vi "InitializeInstrument.vi"(8 "error in (no error)":errorcluster, 11 "reference in":refnum<class "niMmWave_Reciever.lvclass">) -> (0 "error out":errorcluster, 3 "reference out":refnum<class "niMmWave_Reciever.lvclass">)   [LabVIEW 2019, in "niMmWave_Reciever.lvclass"]
doc: "Opens instrument session(s) and performs initial configuration for selected mode.\n\nInputs:\n<b>Initialization source</b> ini file and ini section to be read\n<b>Mode</b> specifies operation mode: BB/IF/RF"
uses:
  niMmWave_Reciever.lvclass
  C:/Barkhausen mmWave radar/Development/modules/mmw_instrument/src_LabVIEW/Host/SubVIs/mmWave instrument_class/mmWave instrument.lvclass
  Low-level/TypeDefs/Resources.ctl
  <vilib>/userdefined/High Color/nirio_resource_hc.ctl
  mmWave instrument_class/Instrument state.ctl
  Low-level/TypeDefs/Hardware Configuration.ctl
  Low-level/TypeDefs/Direction.ctl
  mmWave HW Control/mmWave HW Control.lvlib
  mmWave instrument_class/mmWave instrument.lvclass
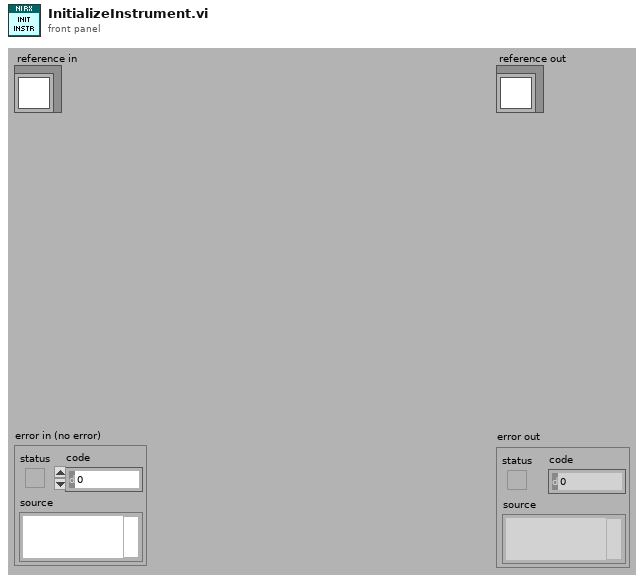
[diagram p1: front panel]
types:
  T1 = typedef "mmWave instrument.lvclass/Instrument state.ctl" = enum16{"Off", "Initialization", "Configuration", "Running", "Calibration"}
  T2 = typedef "Resources.ctl" = cluster{"7902R (Tx)":T3, "3610 (Tx)":refnum<visa-resource-name>, "3620 (IF)":T3, "3630 (RX)":refnum<visa-resource-name>, "7902R (Rx)":T3}
  T3 = typedef "nirio_resource_hc.ctl" = tag
  T4 = typedef "mmWave instrument.lvclass/ObjectAttributesRef.ctl" = refnum<data-value>
  T5 = typedef "niMmWave_Reciever.lvclass/ObjectAttributesRef.ctl" = refnum<data-value>
  T6 = typedef "niMmWave_Reciever.lvclass/ObjectAttributes.ctl" = cluster{"session":T7[], "HW.RX devices":T21, "RF config":T22, "RX trigger options":T23, "RX samples":i32, "RX Fs":dbl}
  T7 = typedef "Session.ctl" = cluster{"3620 session":refnum<queue>, "tx baseband session":T8, "rx baseband session":T16, "tx gain (dB)":dbl, "rx gain (dB)":dbl, "hardware configuration":T17, "gain ranging":T19[], "pxi trigger bus information":T20}
  T8 = typedef "Tx Baseband Session.ctl" = cluster{"3610 session":T9, "7902 reference":T15}
  T9 = typedef "ni3610_and_ni3630_Driver_Lib.lvlib/Main Settings.ctl" = cluster{"VISA resource name":refnum<visa-resource-name>, "Address Space":T10, "window_offset":u32, "register_addresses":T11, "required_MM_fpga_version":cluster{"signature":u32, "hardware":u32, "current revision":u32, "oldest revision":u32}, "CPLD Oldest Compat Version ":cluster{"hardware":u32, "CPLD firmware":u32}, "MM_FPGA_image_location":string, "is_init":bool, "card_type":T12, "DacLmkConfigFileName":string, "AdcLmkConfigFileName":string, "AdcConfigFileName":string, "DacConfigFileName_RevA":string, "DacConfigFileName_RevB":string, "Mulde hardware revision":u8, "bypass DAC PLL\n":bool, "IQ Card Revision":T13, "board capability":T14}
  T10 = typedef "VISA Register Access Address Space.ctl" = u16
  T11 = typedef "ni3610_and_ni3630_Driver_Lib.lvlib/Register Adresses.ctl" = cluster{"MM based Registers":cluster{"Revision":u32, "OldestCompatRev":u32, "signature":u32, "scratch":u32, "LedControl":u32, "BoardHwRev":u32, "BoardControl":u32, "ThermalStatus":u32, "BasebandStatus":u32, "BasebandControl":u32, "BasebandAuxSetup":u32, "BasebandAuxStatus":u32, "LmkSyncOutSetup":u32, " AdcSyncOutSetup":u32, " InjSyncOutSetup":u32, " PxiTrig0OutSetup":u32, " PxiTrig1OutSetup":u32, " PxiTrig2OutSetup":u32, " PxiTrig3OutSetup":u32, " PxiTrig4OutSetup":u32, " PxiTrig5OutSetup":u32, " PxiTrig6OutSetup":u32, " PxiTrig7OutSetup":u32}, "CPLD based Registers":cluster{"SlaveSignature":u32, "SlaveRevision":u32, "SlaveOldestCompatRev":u32, "SlaveScratch":u32, "SlaveSetup":u32, "SlaveStatus":u32, "IDacReg_offset":u32, "LMKRegGrp0_offset":u32, "QDacReg_offset":u32, "BrdTempSensorVal":u32, "TempSensorPowerDown":u32, "GPIOReg_offset":u32, "IAdcReg_offset":u32, "QAdcReg_offset":u32, "LMKRegGrp1_offset":u32, "QadcTempSensorVal":u32, "IadcTempSensorVal":u32, "RevisionReg":u32, "VcxoReg":u32, "CpldStatusReg":u32, "PowerReg":u32, "VBiasEnReg":u32, "ExtRefOeReg":u32, "QdacCtrlReg":u32, "QdacStatusReg":u32, "IdacCtrlReg":u32, "IdacStatusReg":u32, "QdacJtagIn":u32, "QdacJtagOut":u32, "IdacJtagIn":u32, "IdacJtagOut":u32, "IqDcSetupReg":u32, "QadcStatusReg":u32, "IadcStatusReg":u32, "BrdSetupReg":u32, "IqDcRevisionReg":u32, "PllStatusReg":u32, "EndpointScratchReg":u32, "AdcSyncCfgReg":u32, "IqCardOpampReg":u32}, "CPLD Register Offset":u32, "MM  Register Offset":u32, " PxiTrig0OutSetup":u32}
  T12 = typedef "ni3610_and_ni3630_Driver_Lib.lvlib/Base Card Type.ctl" = enum16{"unspecified", "ADC", "DAC"}
  T13 = typedef "ni3610_and_ni3630_Driver_Lib.lvlib/IQ Card Revision.ctl" = enum16{"RevA", "RevB", "RevC", "RevD"}
  T14 = typedef "ni3610_and_ni3630_Driver_Lib.lvlib/Board Capability.ctl" = cluster{"baseband sync":enum16{"no baseband sync", "baseband sync"}}
  T15 = typedef "Blank FPGA Reference.ctl" = refnum<k20>
  T16 = typedef "Rx Baseband Session.ctl" = cluster{"3630 session":T9, "7902 reference":T15}
  T17 = typedef "Hardware Configuration.ctl" = cluster{"direction":T18, "baseband only":bool}
  T18 = typedef "Direction.ctl" = enum16{"Transceiver", "Receiver", "Transmitter"}
  T19 = typedef "Gain Ranging.ctl" = cluster{"gain ranging active scope":string, "gain ranging stream session":refnum<k20>}
  T20 = typedef "PXI Trigger Bus Info.ctl" = cluster{"chassis resource name":refnum<visa-resource-name>, "7902R (TX)":i16, "3610 (TX)":i16, "3620 (IF)":i16, "3630 (RX)":i16, "7902R (RX)":i16}
  T21 = typedef "mmWave HW Control.lvlib/HW RX resources cluster.ctl" = cluster{"HW.IF":tag, "HW.ADC":refnum<visa-resource-name>, "HW.RX FPGA":tag}
  T22 = typedef "mmWave HW Control.lvlib/HW RX RF config cluster.ctl" = cluster{"Gain":dbl, "Frequency":dbl, "mmWave adapter":string}
  T23 = typedef "TX trigger config.ctl" = cluster{"delay":dbl, "trig source":T24, "PXI src":i32, "export":T25, "PXI dest":i32}
  T24 = typedef "FPGA Utility.lvlib/FPGA driver trigger source.ctl" = enum16{"Use Tclk", "PXI_Trig", "Aurora RX trig"}
  T25 = typedef "FPGA Utility.lvlib/FPGA driver trigger destination.ctl" = enum16{"None", "Source trig", "Synced trig", "Delayed sync"}
  T26 = typedef "mmWave instrument.lvclass/ObjectAttributes.ctl" = cluster{"mode":T27, "instr state":T1, "Max Fs":dbl, "Equalization coeff":cdb[], "LO sync en":bool, "Trig sync en":bool, "LO sources":T28, "LO Export":T29, "Fc.range":cluster{"min":dbl, "max":dbl}, "Sync mode":T30, "equalization en":bool, "sequence":string[]}
  T27 = typedef "mmWave instrument.lvclass/Instrument mode.ctl" = enum16{"RF", "IF", "BB"}
  T28 = typedef "mmWave HW Control.lvlib/LO sources.ctl" = cluster{"RX/LO1 src":string, "TX/LO1 src":string, "LO2 src":string}
  T29 = typedef "mmWave HW Control.lvlib/LO export.ctl" = cluster{"TX LO1 export":bool, "TX LO1 export level":dbl, "RX LO1 export":bool, "RX LO1 export level":dbl, "LO2 export":bool, "LO2 export level":dbl}
  T30 = typedef "mmWave instrument.lvclass/Sync mode.ctl" = enum16{"Slave", "Master"}
  T31 = typedef "Detected mmWave Adapters.ctl" = cluster{"3620 resource name":T3, "detected mmWave adapters":T32[]}
  T32 = typedef "mmWave Adapter Information.ctl" = cluster{"scope":string, "mmWave adapter type":string, "serial number":u64}
  T33 = typedef "Constants.ctl" = cluster{"data clock rate (Hz)":dbl, "sample rate (Hz)":dbl, "sample rate selector string":string, "default tx bitfile path":path, "default rx bitfile path":path, "default proc bitfile path":path}
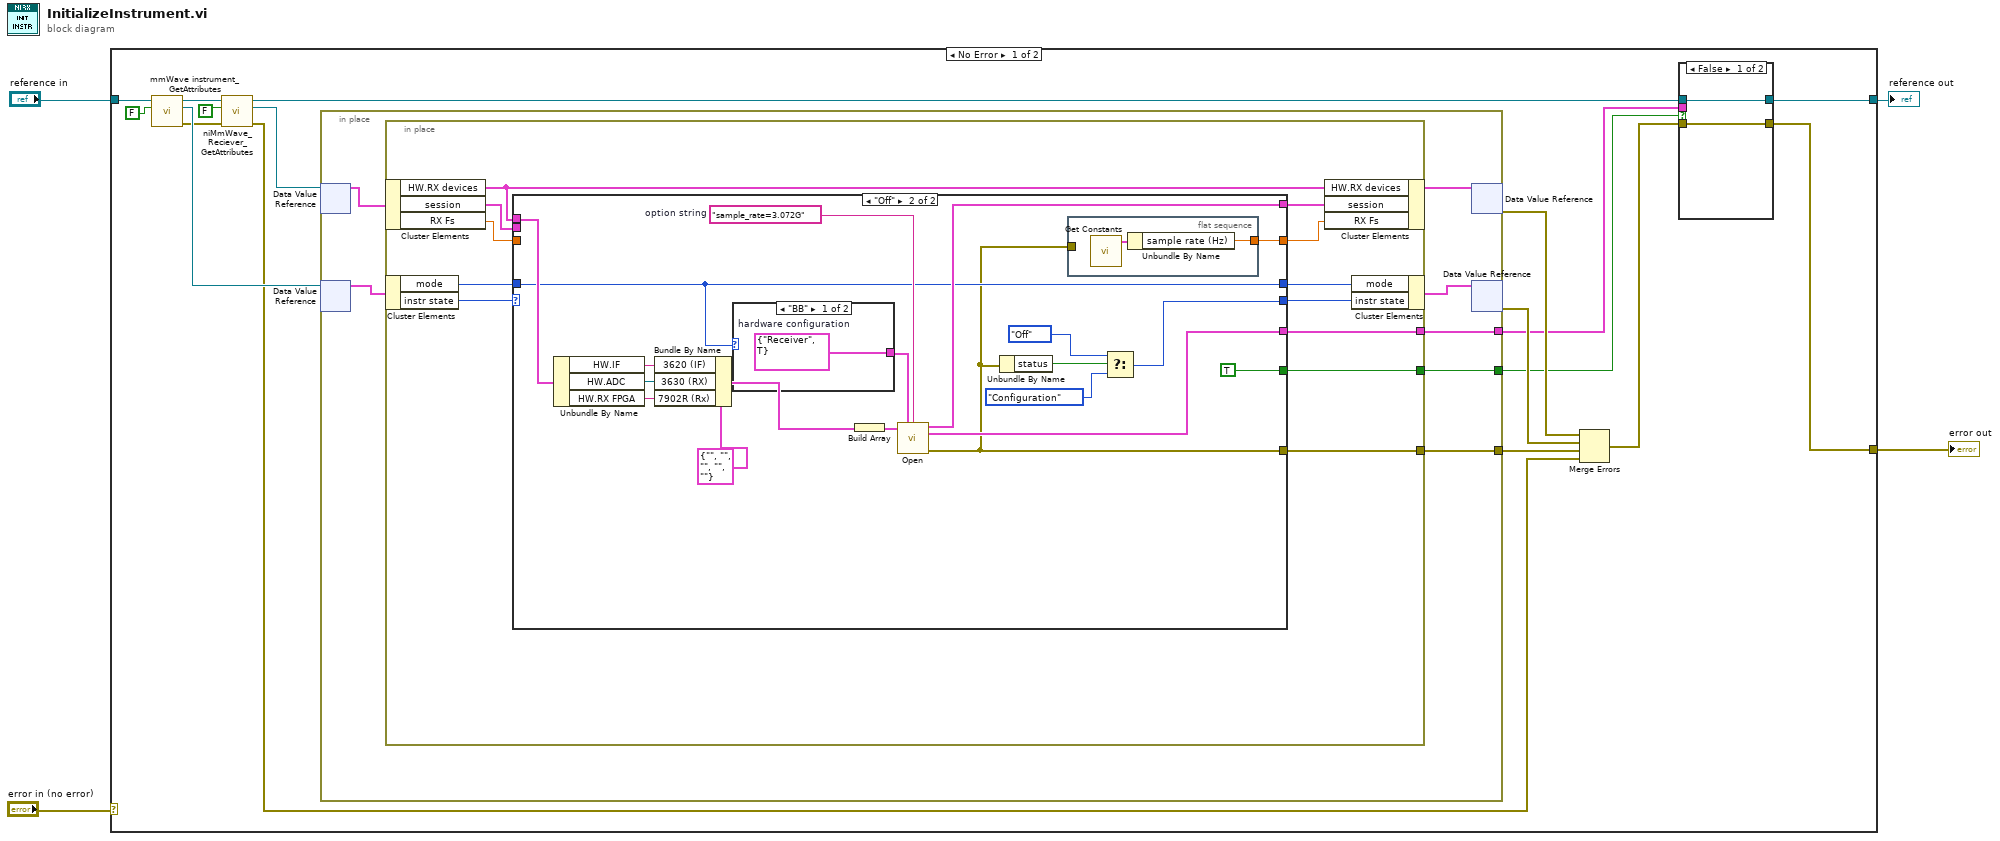
[diagram p0: block diagram]
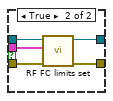
[diagram p2: hidden frame]
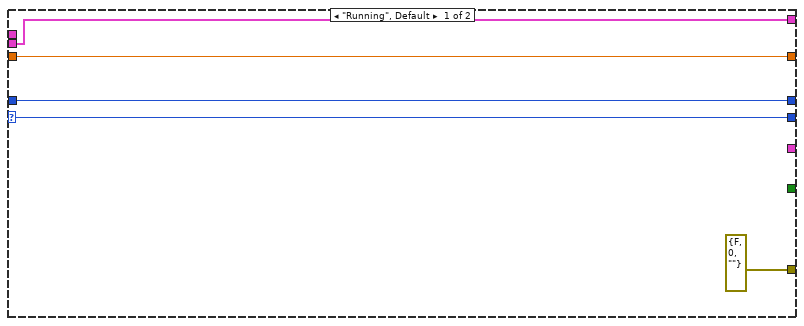
[diagram p3: hidden frame]
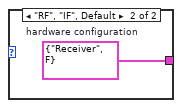
[diagram p4: hidden frame]
diagram:
  n1 = case shown="No Error" "error in (no error)" {
    selector: "error in (no error)" -> [_ w77]
    tunnel: [w6 w77] -> w3
    tunnel: [w9 w76] -> w1
    tunnel: "reference in" -> [w20 w76]
    frame No Error {
      n2 = call "mmWave instrument_GetAttributes.vi"("return data? (T)"=FALSE, "reference in"=w20) -> ("error out"=w13:errorcluster, "attributes ref"=w15:T4, "reference out"=w19:refnum<class "niMmWave_Reciever.lvclass">)  [unwired: 6 in, 1 out]
      n3 = call "niMmWave_Reciever_GetAttributes.vi"("error in (no error)"=w13, "return data? (T)"=FALSE, "reference in"=w19) -> ("error out"=w10:errorcluster, "attributes ref"=w16:T5, "reference out"=w21:refnum<class "niMmWave_Reciever.lvclass">)  [unwired: 5 in, 1 out]
      n4 = in-place {
        in-place-border: [w31] -> w14
        in-place-border: [w30] -> w8
        in-place-border: [w29] -> w5
        n5 = in-place-dvr #1(w16) -> (w35:T6)  [unwired: 1 out]
        n6 = in-place-dvr #2(w15) -> (w33:T26)  [unwired: 1 out]
        n7 = in-place {
          in-place-border: [w44] -> w31
          in-place-border: [w38] -> w30
          in-place-border: [w37] -> w29
          n8 = in-place-cluster #3(w35) -> ("HW.RX devices"=w47:T21, "session"=w36:T7[], "RX Fs"=w39:dbl)
          n9 = in-place-cluster #4(w33) -> ("mode"=w45:T27, "instr state"=w42:T1)
          n10 = case shown="\"Off\"" w42 {
            selector: w42 -> [w48 _]
            tunnel: w47 -> [_ w64]
            tunnel: [w49 w63] -> w46
            tunnel: w45 -> [w52 w57]
            tunnel: [errorcluster {"status"=FALSE, "code"=0, "source"=""} ("error out") w53] -> w44
            tunnel: [w48 w58] -> w43
            tunnel: [w52 w57] -> w41
            tunnel: [w50 w56] -> w40
            tunnel: w39 -> [w50 _]
            tunnel: [_ w55] -> w38
            tunnel: [_ TRUE] -> w37
            tunnel: w36 -> [w49 _]
            frame "Running", Default {
            }
            frame "Off" {
              w65 = "sample_rate=3.072G"  # option string
              n11 = Unbundle By Name(w64) -> ("HW.IF"=w69:tag, "HW.ADC"=w68:refnum<visa-resource-name>, "HW.RX FPGA"=w67:tag)
              n12 = Bundle By Name(cluster=T2 {"7902R (Tx)"="", "3610 (Tx)"="", "3620 (IF)"="", "3630 (RX)"="", "7902R (Rx)"=""} ("resources"), "3620 (IF)"=w69, "3630 (RX)"=w68, "7902R (Rx)"=w67) -> (w71:T2)
              n13 = case shown="\"BB\"" w57 {
                tunnel: [w74 w75] -> w62
                frame "BB" {
                  w74 = T17 {"direction"=enum."Receiver", "baseband only"=TRUE}  # hardware configuration
                }
                frame "RF", "IF", Default {
                  w75 = T17 {"direction"=enum."Receiver", "baseband only"=FALSE}  # hardware configuration
                }
              }
              n14 = Build Array(w71) -> (w70:T2[])
              n15 = call "Open.vi"("resources"=w70, "hardware configuration"=w62, "option string"=w65) -> ("session out"=w63:T7[], "detected mmWave adapters"=w55:T31[], "error out"=w53:errorcluster)  [unwired: 10 in]
              n16 = Unbundle By Name(w53) -> ("status"=w61:bool)
              n17 = flat-sequence {
                tunnel: [w73] -> w56
                tunnel: w53 -> [_]
                frame #0 {
                  n18 = call "Get Constants.vi"() -> ("constants"=w72:T33)  [unwired: 15 in]
                  n19 = Unbundle By Name(w72) -> ("sample rate (Hz)"=w73:dbl)
                }
              }
              n20 = Select(t=Instrument_state."Off" ("instr state"), s=w61, f=Instrument_state."Configuration" ("instr state")) -> (s? t:f=w58:T1)
            }
          }
          n21 = in-place-cluster #3("HW.RX devices"=w47, "session"=w46, "RX Fs"=w40) -> (w34:T6)
          n22 = in-place-cluster #4("mode"=w41, "instr state"=w43) -> (w32:T26)
        }
        n23 = in-place-dvr #1(w34) -> (w12:errorcluster)  [unwired: 1 out]
        n24 = in-place-dvr #2(w32) -> (w11:errorcluster)  [unwired: 1 out]
      }
      n25 = Merge Errors(w12, w11, w14, w10) -> (w7:errorcluster)
      n26 = case shown="False" w5 {
        tunnel: w21 -> [w23 w28]
        tunnel: [w23 w27] -> w9
        tunnel: w8 -> [_ w26]
        tunnel: w7 -> [w22 w25]
        tunnel: [w22 w24] -> w6
        frame False {
        }
        frame True {
          n27 = call-dynamic "RF FC limits set.vi"("error in (no error)"=w25, "detected mmWave adapters"=w26, "reference in"=w28) -> ("error out"=w24:errorcluster, "reference out"=w27:refnum<class "niMmWave_Reciever.lvclass">)  [unwired: 7 in]
        }
      }
    }
    frame Error {
    }
  }
  "error out" <- w3
  "reference out" <- w1
